vi "Configure Averaging.vi"(7 "Enable Averaging (T: Enable)":bool=TRUE, 8 "error in (no error)":errorcluster, 9 "Averaging Type (0: Auto)":u16(ring) items=["Auto", "RMS", "Video", "Scalar"], 10 "Average Count (100)":i32=100, 11 "VISA resource name":refnum<visa-resource-name>) -> (0 "error out":errorcluster, 3 "VISA resource name out":refnum<visa-resource-name>)   [LabVIEW 2014, in "Agilent ESA PSA Series.lvlib"]
doc: "Configures the averaging."
uses:
  Agilent ESA PSA Series.lvlib
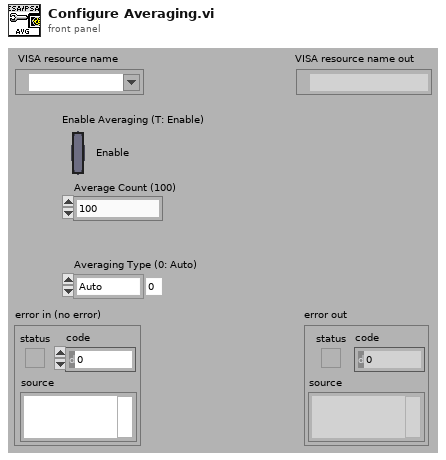
[diagram p1: front panel]
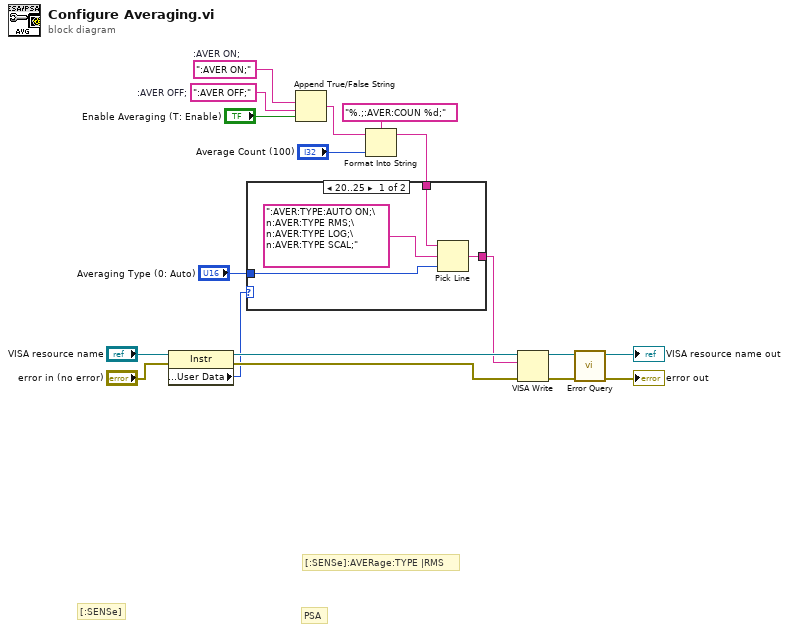
[diagram p0: block diagram]
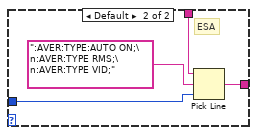
[diagram p2: hidden frame]
diagram:
  w3 = ":AVER OFF;"  # :AVER OFF;
  w13 = ":AVER ON;"  # :AVER ON;
  # "PSA"
  # "[:SENSe]:AVERage:TYPE |RMS"
  # "[:SENSe]"
  n1 = property on="Property Node" class="Instr"(reference="VISA resource name", error in="error in (no error)") -> (reference out=w7:refnum<visa-resource-name>, error out=w6:errorcluster, "General Settings:User Data"=w5:u32)
  n2 = Append True/False String(1:"Enable Averaging (T: Enable)", 2:w3, 3:w13) -> (0:w2:string)  [unwired: 1 in]
  n3 = Format Into String(format string="%.;:AVER:COUN %d;", initial string=w2, "Average Count (100)") -> (resulting string=w1:string)  [unwired: 1 in, 1 out]
  n4 = case shown="20..25" w5 {
    tunnel: [w22 w26] -> w4
    tunnel: "Averaging Type (0: Auto)" -> [w21 w25]
    tunnel: w1 -> [w19 w23]
    frame 20..25 {
      n5 = Pick Line(string ("")=w19, multi-line string=":AVER:TYPE:AUTO ON;\n:AVER:TYPE RMS;\n:AVER:TYPE LOG;\n:AVER:TYPE SCAL;", line index=w21) -> (output string=w22:string)
    }
    frame Default {
      # "ESA"
      n6 = Pick Line(string ("")=w23, multi-line string=":AVER:TYPE:AUTO ON;\n:AVER:TYPE RMS;\n:AVER:TYPE VID;", line index=w25) -> (output string=w26:string)
    }
  }
  n7 = VISA Write(VISA resource name=w7, write buffer=w4, error in (no error)=w6) -> (VISA resource name out=w17:refnum<visa-resource-name>, error out=w15:errorcluster)  [unwired: 1 out]
  n8 = call "Error Query.vi"("error in (no error)"=w15, "VISA resource name"=w17) -> ("error out"=→"error out":errorcluster, "VISA resource name out"=→"VISA resource name out":refnum<visa-resource-name>)  [unwired: 6 in, 2 out]
